vi "Output External Query.vi"(8 "error in":errorcluster, 11 "Instrument Handle In":i32) -> (0 "error out":errorcluster, 1 "Source":i32, 2 "State":i32, 3 "Instrument Handle Out":i32, 4 "Polarity":i32, 5 "Pulse Period":dbl, 6 "Pulse Mode":i32)   [LabVIEW 8.6, in "ZTScopeM.lvlib"]
doc: "Query the external output configuration."
uses:
  ZTScopeM.lvlib
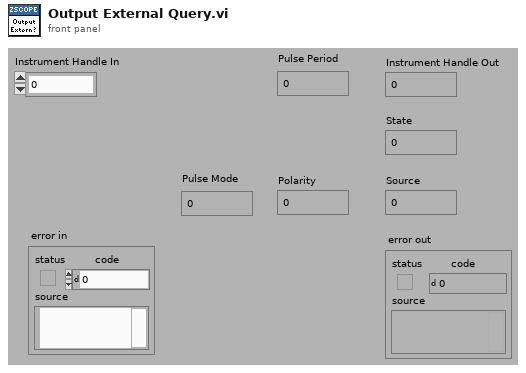
[diagram p1: front panel]
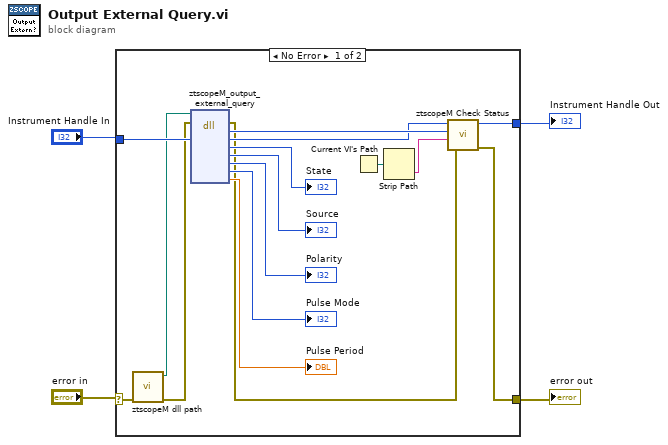
[diagram p0: block diagram]
diagram:
  n1 = case shown="No Error" "error in" {
    selector: "error in" -> [w8 w22]
    tunnel: [w9 w22] -> w2
    tunnel: "Instrument Handle In" -> [w20 w21]
    tunnel: [w10 w21] -> w4
    frame #0 {
      n2 = call "ztscopeM dll path.vi"("error in (no error)"=w8) -> ("error out"=w6:errorcluster, "<instrument>.dll path"=w7:path)  [unwired: 9 in]
      n3 = dll-call lib="C:/Program Files (x86)/National Instruments/LabVIEW 2013/instr.lib/ztscopem/ztscopeM.dll" fn="ztscopeM_output_external_query"(path in=w7, error in=w6, "instrumentHandle"=w20) -> (error out=w5:errorcluster, w12:i32, "instrumentHandle"=w11:i32, "state"=→"State":i32, "source"=→"Source":i32, "polarity"=→"Polarity":i32, "pulseMode"=→"Pulse Mode":i32, "pulsePeriod"=→"Pulse Period":dbl)  [unwired: 6 in, 1 out]
      n4 = Current VI's Path() -> (path=w14:path)
      n5 = Strip Path(path=w14) -> (name=w13:string)  [unwired: 1 out]
      n6 = call "ztscopeM Check Status.vi"("error in"=w5, "name of VI"=w13, "status (return code)"=w12, "instrument handle in"=w11) -> ("error out"=w9:errorcluster, "instrument handle out"=w10:i32)  [unwired: 2 in]
    }
    frame #1 {
    }
  }
  "Instrument Handle Out" <- w4
  "error out" <- w2
